vi "GetGraphicsAndContainer.vi"(0 "LcPictureBox in":refnum<class "LcPictureBox.lvclass">, 5 "error in (no error)":errorcluster) -> (14 "LcPictureBox out":refnum<class "LcPictureBox.lvclass">, 15 "CreateGraphics":refnum<k24>, 16 "ContinerCreated":bool, 17 "CreatedContainerRef":refnum<k24>, 19 "error out":errorcluster)   [LabVIEW 2019, in "LcPictureBox.lvclass"]
uses:
  LcPictureBox.lvclass
  System.Drawing
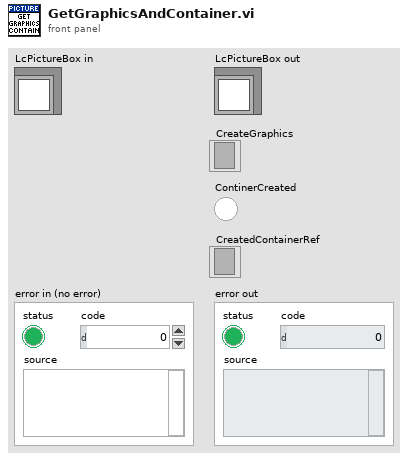
[diagram p1: front panel]
types:
  T1 = typedef "LcPictureBox.lvclass/ObjectAttributes.ctl" = cluster{"PictureBox":refnum<k24>, "ImageSize(PictureBoxSize)":cluster{"Width":i32, "Height":i32}, "PenMemory":map{cluster{"Alpha(100%)":dbl, "Color(Black)":u32, "Pen(Width=1, Solid)":T2}, refnum<k24>}, "GraphicsRef":refnum<k24>, "BrushMemory":map{cluster{"Alpha(100%)":dbl, "Color(Black)":u32}, refnum<k24>}, "Containers":refnum<k24>[], "Images":refnum<k24>[]}
  T2 = typedef "LcPictureBox.lvclass/Pen.ctl" = cluster{"Width":u16, "Style":enum32{"Solid", "Dash", "Dot", "DashDot", "DashDotDot"}}
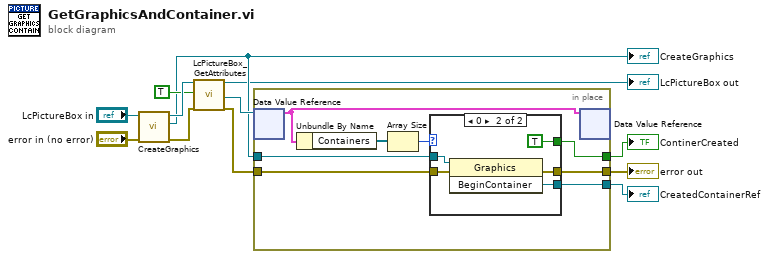
[diagram p0: block diagram]
diagram:
  n1 = call "CreateGraphics.vi"("error in (no error)"="error in (no error)", "LcPictureBox in"="LcPictureBox in") -> ("error out"=w11:errorcluster, "CreateGraphics"=w3:refnum<k24>, "LcPictureBox out"=w10:refnum<class "LcPictureBox.lvclass">)  [unwired: 7 in]
  "CreateGraphics" <- w3
  n2 = call "LcPictureBox_GetAttributes.vi"("reference in"=w10, "OnlyGetDvrReference(False)"=TRUE, "error in (no error)"=w11) -> ("reference out"=→"LcPictureBox out":refnum<class "LcPictureBox.lvclass">, "DataRef"=w8:refnum<data-value>, "error out"=w12:errorcluster)  [unwired: 13 in, 1 out]
  n3 = in-place {
    in-place-border: w3 -> [w20]
    in-place-border: w12 -> [w18]
    in-place-border: [w17] -> w2
    in-place-border: [w14] -> w5
    in-place-border: [w13] -> w4
    n4 = in-place-dvr #1(w8) -> (w15:T1)  [unwired: 1 out]
    n5 = Unbundle By Name(w15) -> ("Containers"=w19:refnum<k24>[])
    n6 = Array Size(array=w19) -> (size(s)=w16:i32)
    n7 = case shown="0" w16 {
      tunnel: w20 -> [_ w26]
      tunnel: w18 -> [w21 w25]
      tunnel: [w21 w24] -> w17
      tunnel: [_ w23] -> w14
      tunnel: [_ TRUE] -> w13
      frame 1.., Default {
      }
      frame 0 {
        n8 = invoke class="Graphics" method="BeginContainer"(reference=w26, error in=w25) -> (error out=w24:errorcluster, "BeginContainer"=w23:refnum<k24>)  [unwired: 1 in, 1 out]
      }
    }
    n9 = in-place-dvr #1(w15) -> ()  [unwired: 2 out]
  }
  "error out" <- w2
  "ContinerCreated" <- w4
  "CreatedContainerRef" <- w5
